vi "Panel Resized.vi"(6 "Sizing Refnums":T2, 8 "error in (no error)":errorcluster, 9 "Origin":cluster{"H":i16, "V":i16}, 10 "NewBnds":T1, 11 "Size Constraints":cluster{"min tab width":i32, "w/h":dbl}) -> (0 "error out":errorcluster)   [LabVIEW 2016]
uses:
  <vilib>/Utility/miscctls.llb/LVRectTypeDef.ctl
  <vilib>/Utility/miscctls.llb/LVRowAndColumnTypeDef.ctl
panel:
  out "Array":cluster{u32, u32}[](array[cluster])
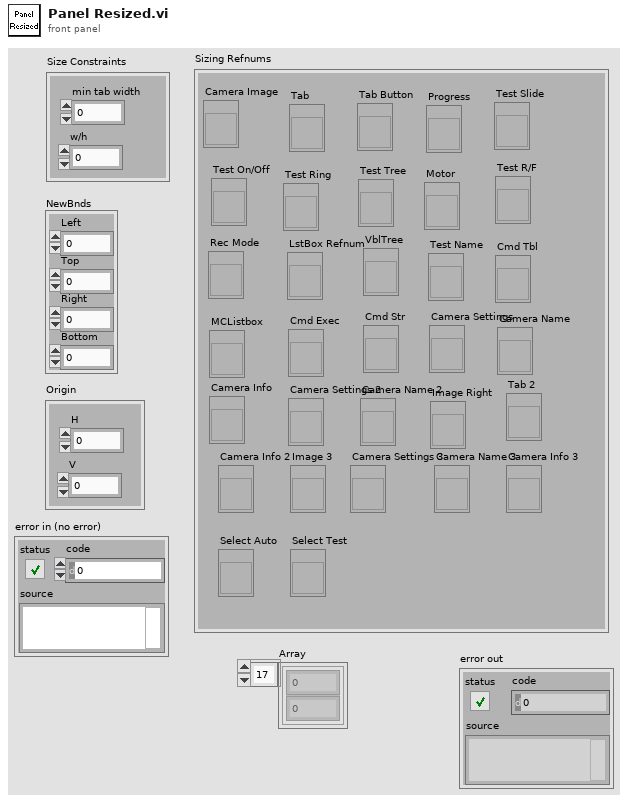
[diagram p1: front panel]
types:
  T1 = typedef "LVRectTypeDef.ctl" = cluster{"Left":i16, "Top":i16, "Right":i16, "Bottom":i16}
  T2 = cluster{"Camera Image":refnum<vi>, "Tab":refnum<vi>, "Tab Button":refnum<vi>, "Rec Mode":refnum<vi>, "Test Slide":refnum<vi>, "Test On/Off":refnum<vi>, "Test Ring":refnum<vi>, "Test R/F":refnum<vi>, "Test Name":refnum<vi>, "Motor":refnum<vi>, "Progress":refnum<vi>, "LstBox Refnum":refnum<vi>, "Test Tree":refnum<vi>, "VblTree":refnum<vi>, "Cmd Tbl":refnum<vi>, "MCListbox":refnum<vi>, "Cmd Exec":refnum<vi>, "Cmd Str":refnum<vi>, "Camera Settings":refnum<vi>, "Camera Name":refnum<vi>, "Camera Info":refnum<vi>, "Camera Settings 2":refnum<vi>, "Camera Name 2":refnum<vi>, "Image Right":refnum<vi>, "Tab 2":refnum<vi>, "Camera Info 2":refnum<vi>, "Image 3":refnum<vi>, "Camera Settings 3":refnum<vi>, "Camera Name 3":refnum<vi>, "Camera Info 3":refnum<vi>, "Select Auto":refnum<vi>, "Select Test":refnum<vi>}
  T3 = typedef "LVRowAndColumnTypeDef.ctl" = cluster{"Row":i32, "Column":i32}
  T4 = typedef "LVBoundsTypeDef.ctl" = cluster{"Width":u32, "Height":u32}
  T5 = typedef "LVPositionTypeDef.ctl" = cluster{"Left":i32, "Top":i32}
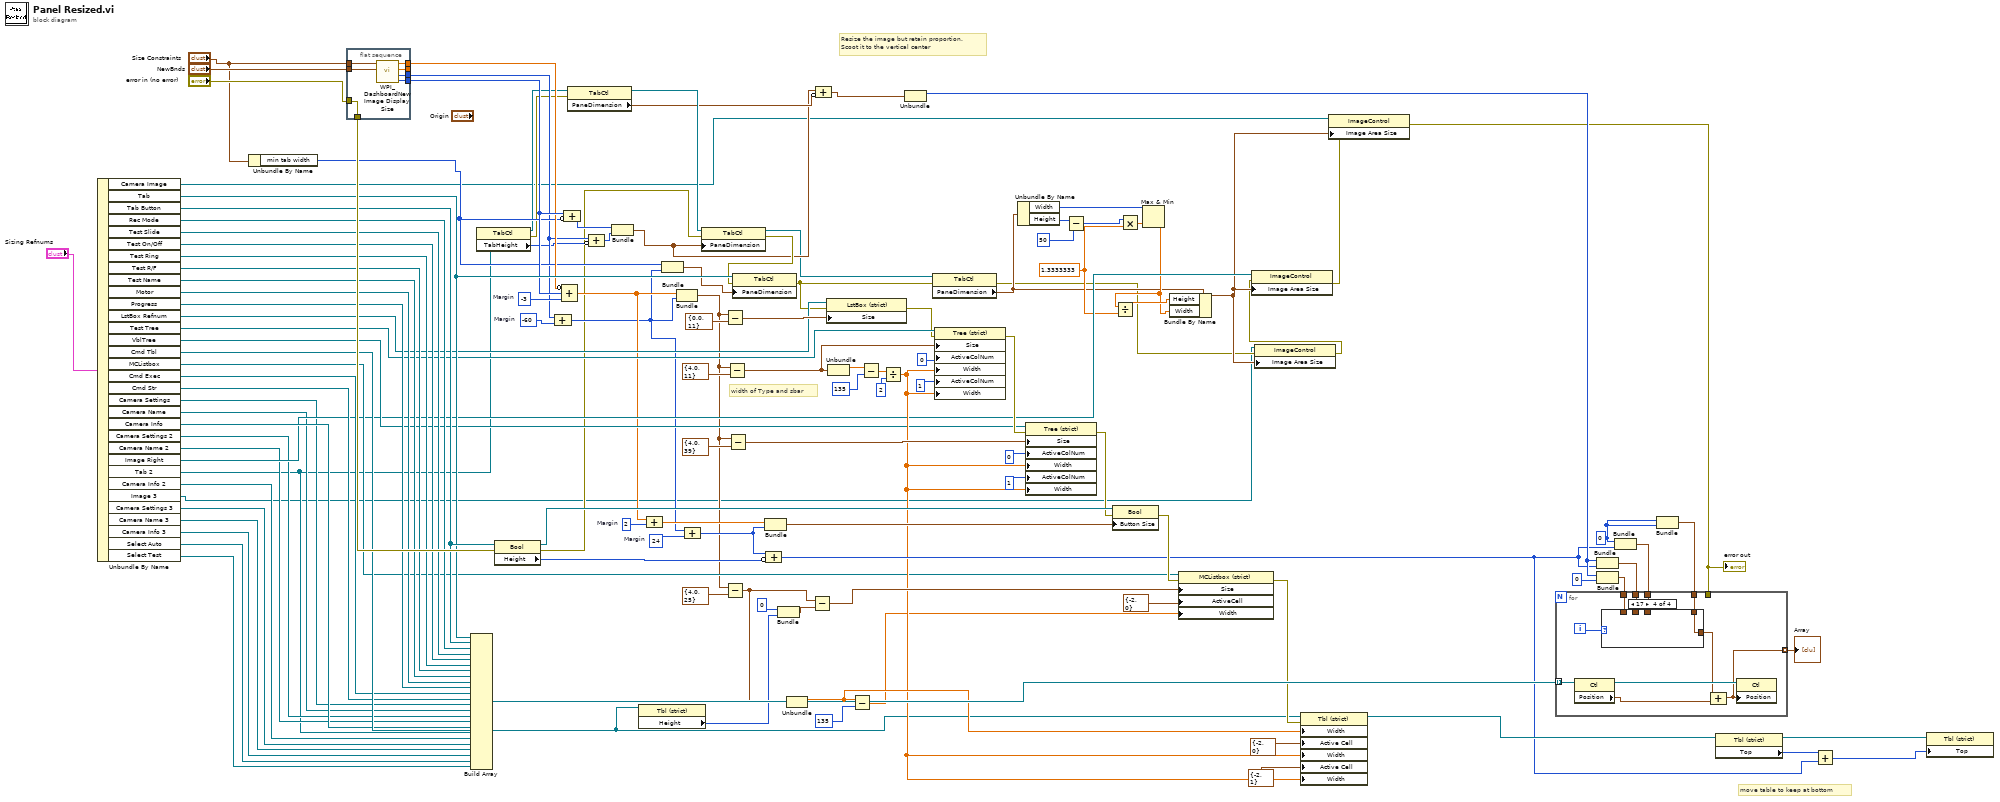
[diagram p0: block diagram]
diagram:
  w44 = 1.3333333 ("y")
  w41 = 0
  w120 = 24  # Margin
  w119 = 2  # Margin
  w19 = -60  # Margin
  w28 = -3  # Margin
  # "move table to keep at bottom"
  # "width of Type and sbar"
  # "Resize the image but retain proportion.\nScoot it to the vertical center"
  n1 = Unbundle By Name("Sizing Refnums") -> ("Camera Image"=w10:refnum<vi>, "Tab"=w109:refnum<vi>, "Tab Button"=w114:refnum<vi>, "Rec Mode"=w71:refnum<vi>, "Test Slide"=w70:refnum<vi>, "Test On/Off"=w69:refnum<vi>, "Test Ring"=w68:refnum<vi>, "Test R/F"=w67:refnum<vi>, "Test Name"=w66:refnum<vi>, "Motor"=w65:refnum<vi>, "Progress"=w64:refnum<vi>, "LstBox Refnum"=w63:refnum<vi>, "Test Tree"=w62:refnum<vi>, "VblTree"=w61:refnum<vi>, "Cmd Tbl"=w60:refnum<vi>, "MCListbox"=w59:refnum<vi>, "Cmd Exec"=w58:refnum<vi>, "Cmd Str"=w57:refnum<vi>, "Camera Settings"=w33:refnum<vi>, "Camera Name"=w32:refnum<vi>, "Camera Info"=w56:refnum<vi>, "Camera Settings 2"=w31:refnum<vi>, "Camera Name 2"=w30:refnum<vi>, "Image Right"=w55:refnum<vi>, "Tab 2"=w16:refnum<vi>, "Camera Info 2"=w34:refnum<vi>, "Image 3"=w1:refnum<vi>, "Camera Settings 3"=w9:refnum<vi>, "Camera Name 3"=w8:refnum<vi>, "Camera Info 3"=w7:refnum<vi>, "Select Auto"=w6:refnum<vi>, "Select Test"=w5:refnum<vi>)
  n2 = Unbundle By Name("Size Constraints") -> ("min tab width"=w25:i32)
  n3 = flat-sequence {
    tunnel: "NewBnds" -> [w134]
    tunnel: "Size Constraints" -> [w133]
    tunnel: [w132] -> w43
    tunnel: [w131] -> _
    tunnel: [w130] -> w17
    tunnel: [w129] -> w35
    tunnel: [w128] -> w126
    tunnel: "error in (no error)" -> [w128]
    frame #0 {
      n4 = call <vilib>:"WPI_DashboardNew Image Display Size.vi"("NewBnds"=w134, "Size Constraints"=w133) -> ("Window Width"=w132:i16, "Window Height"=w130:i16, "Height"=w131:dbl, "Width"=w129:dbl)  [unwired: 6 in]
    }
  }
  n5 = Build Array(w109, w114, w71, w70, w69, w68, w67, w66, w65, w64, w58, w57, w33, w32, w31, w30, w56, w16, w34, w9, w8, w7, w6, w5) -> (w127:refnum<vi>[])
  n6 = property class="TabCtl"(reference=w16) -> (reference out=w14:refnum<vi>, error out=w13:errorcluster, "TabHeight"=w15:u32)  [unwired: 1 in]
  n7 = property class="Bool"(reference=w114, error in=w126) -> (reference out=w123:refnum<vi>, error out=w11:errorcluster, "Height"=w122:u32)
  n8 = Compound Arithmetic op=unknown(w17, w19) -> (w12:i32)
  n9 = Compound Arithmetic op=ADD(invert w35, w43, w28) -> (w51:dbl)
  n10 = Compound Arithmetic op=ADD(w43, invert w25) -> (w42:i32)
  n11 = property class="TabCtl"(reference=w14, error in=w13) -> (reference out=w39:refnum<vi>, "PaneDimension"=w38:T4)  [unwired: 1 out]
  n12 = Compound Arithmetic op=ADD(w17, invert w15) -> (w18:u32)
  n13 = Bundle(w42, w18) -> (w37:cluster{i32, u32})  [unwired: 1 in]
  n14 = property class="Tbl (strict)"(reference=w60) -> ("Height"=w87:u32)  [unwired: 1 in, 2 out]
  n15 = Compound Arithmetic op=ADD(w51, w119) -> (w118:dbl)
  n16 = Bundle("min tab width"=w25, w12) -> (w52:cluster{"min tab width":i32, i32})  [unwired: 1 in]
  n17 = Bundle(w51, w12) -> (w53:cluster{dbl, i32})  [unwired: 1 in]
  n18 = Compound Arithmetic op=ADD(w12, w120) -> (w121:i32)
  n19 = property class="TabCtl"(reference=w39, error in=w11, "PaneDimension"=w37) -> (reference out=w23:refnum<vi>, error out=w54:errorcluster)
  n20 = Subtract(x=w53, y=cluster{dbl, i32} {0.0, 11}) -> (x-y=w108:cluster{dbl, i32})
  n21 = Subtract(x=w53, y=cluster{dbl, i32} {4.0, 25}) -> (x-y=w84:cluster{dbl, i32})
  n22 = Subtract(x=w53, y=cluster{dbl, i32} {4.0, 11}) -> (x-y=w99:cluster{dbl, i32})
  n23 = Subtract(x=w53, y=cluster{dbl, i32} {4.0, 39}) -> (x-y=w104:cluster{dbl, i32})
  n24 = property class="TabCtl"(reference=w109, error in=w54, "PaneDimension"=w52) -> (error out=w47:errorcluster)  [unwired: 1 out]
  n25 = Bundle(w118, w121) -> (w117:cluster{dbl, i32})  [unwired: 1 in]
  n26 = Compound Arithmetic op=ADD(w121, invert w122) -> (w79:u32)
  n27 = Bundle(0, "Height"=w87) -> (w85:cluster{i32, "Height":u32})  [unwired: 1 in]
  n28 = Unbundle(w84) -> (w75:dbl)  [unwired: 1 out]
  n29 = Subtract(x=w84, y=w85) -> (x-y=w83:cluster{dbl, u32})
  n30 = Compound Arithmetic op=ADD(w37, invert w38) -> (w36:T4)
  n31 = property class="LstBox (strict)"(reference=w63, error in=w47, "Size"=w108) -> (error out=w49:errorcluster)  [unwired: 1 out]
  n32 = Unbundle(w99) -> (w98:dbl)  [unwired: 1 out]
  n33 = Subtract(x=w75, y=135) -> (x-y=w72:dbl)
  n34 = Subtract(x=w98, y=135 ("Active Cell:Active Column Number")) -> (x-y=w94:dbl)
  n35 = Divide(x=w94, y=2 ("Active Cell:Active Column Number")) -> (x/y=w73:dbl)
  n36 = Unbundle(w36) -> ("Width"=w124:u32)  [unwired: 1 out]
  n37 = property class="TabCtl"(reference=w23, error in=w47) -> (error out=w2:errorcluster, "PaneDimension"=w24:T4)  [unwired: 1 out]
  n38 = property class="Tree (strict)"(reference=w62, error in=w49, "Size"=w99, "ActiveColNum"=0 ("Active Cell:Active Column Number"), "Width"=w73, "ActiveColNum"=1 ("Active Cell:Active Column Number"), "Width"=w73) -> (error out=w103:errorcluster)  [unwired: 1 out]
  n39 = Unbundle By Name(w24) -> ("Width"=w46:u32, "Height"=w21:u32)
  n40 = property class="Tree (strict)"(reference=w61, error in=w103, "Size"=w104, "ActiveColNum"=0 ("Active Cell:Active Column Number"), "Width"=w73, "ActiveColNum"=1 ("Active Cell:Active Column Number"), "Width"=w73) -> (error out=w102:errorcluster)  [unwired: 1 out]
  n41 = Subtract(x=w21, y=u32 50) -> (x-y=w22:u32)
  n42 = property class="Bool"(reference=w123, error in=w102, "Button Size"=w117) -> (error out=w91:errorcluster)  [unwired: 1 out]
  n43 = Multiply(x=w22, y=w44) -> (x*y=w45:dbl)
  n44 = Max & Min(x=w46, y=w45) -> (min(x,y)=w26:dbl)  [unwired: 1 out]
  n45 = Divide(x=w26, y=w44) -> (x/y=w27:dbl)
  n46 = Bundle By Name(cluster=w24, "Height"=w27, "Width"=w26) -> (w4:T4)
  n47 = property class="MCListbox (strict)"(reference=w59, error in=w91, "Size"=w83, "ActiveCell"=T3 {"Row"=-2, "Column"=0} ("Active Cell:Active Cell"), "Width"=w72) -> (error out=w88:errorcluster)  [unwired: 1 out]
  n48 = property class="ImageControl"(reference=w1, error in=w2, "Image Area Size"=w4) -> (error out=w3:errorcluster)  [unwired: 1 out]
  n49 = property class="ImageControl"(reference=w55, error in=w3, "Image Area Size"=w4) -> (error out=w48:errorcluster)  [unwired: 1 out]
  n50 = property class="Tbl (strict)"(reference=w60, error in=w88, "Width"=w75, "Active Cell"=T3 {"Row"=-2, "Column"=0} ("Active Cell:Active Cell"), "Width"=w73, "Active Cell"=T3 {"Row"=-2, "Column"=1} ("Active Cell:Active Cell"), "Width"=w73) -> (reference out=w82:refnum<vi>)  [unwired: 1 out]
  n51 = property class="ImageControl"(reference=w10, error in=w48, "Image Area Size"=w4) -> (error out=w112:errorcluster)  [unwired: 1 out]
  "error out" <- w112
  n52 = Bundle("Width"=w124, w79) -> (w116:cluster{"Width":u32, u32})  [unwired: 1 in]
  n53 = Bundle("Width"=w124, 0) -> (w115:cluster{"Width":u32, i32})  [unwired: 1 in]
  n54 = Bundle(w41, w79) -> (w92:cluster{i32, u32})  [unwired: 1 in]
  n55 = Bundle(w41, w41) -> (w40:cluster{i32, i32})  [unwired: 1 in]
  n56 = for {
    tunnel: w127 -> [w144] mode=indexing
    tunnel: w116 -> [w139]
    tunnel: w115 -> [w140]
    tunnel: w112 -> [_]
    tunnel: w92 -> [w138]
    tunnel: w40 -> [w136]
    tunnel: [w135] -> w29 mode=indexing
    i -> [w141]
    n57 = property class="Ctl"(reference=w144) -> (reference out=w143:refnum<vi>, "Position"=w142:T5)  [unwired: 1 in, 1 out]
    n58 = case shown="17" w141 {
      tunnel: w140 -> [_ w146 _ _]
      tunnel: w139 -> [_ _ w147 _]
      tunnel: w138 -> [w145 _ _ _]
      tunnel: [w145 w146 w147 w148] -> w137
      tunnel: w136 -> [_ _ _ w148]
      frame Default {
      }
      frame 0 {
      }
      frame 2..4 {
      }
      frame 17 {
      }
    }
    n59 = Compound Arithmetic op=ADD(w137, w142) -> (w135:cluster{u32, u32})
    n60 = property class="Ctl"(reference=w143, "Position"=w135) -> ()  [unwired: 1 in, 2 out]
  }
  "Array" <- w29
  n61 = property class="Tbl (strict)"(reference=w82) -> (reference out=w81:refnum<vi>, "Top"=w80:i32)  [unwired: 1 in, 1 out]
  n62 = Add(x=w80, y=w79) -> (x+y=w78:u32)
  n63 = property class="Tbl (strict)"(reference=w81, "Top"=w78) -> ()  [unwired: 1 in, 2 out]
